vi "Create IMAQ Img from Channels.vi"(4 "Channel Name(s)":string[](array[string])) -> (0 "IMAQ Ch Images":T1[](array[typedef]), 1 "Channel Name(s) out":string[](array[string]))   [LabVIEW 2020]
uses:
  <vilib>/vision/Image Controls.llb/IMAQ Image.ctl
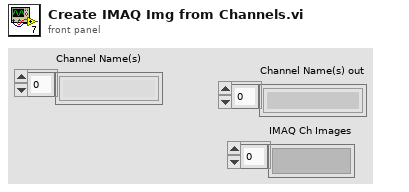
[diagram p1: front panel]
types:
  T1 = typedef "IMAQ Image.ctl" = refnum<image>
  T2 = typedef "Image Type" = u32
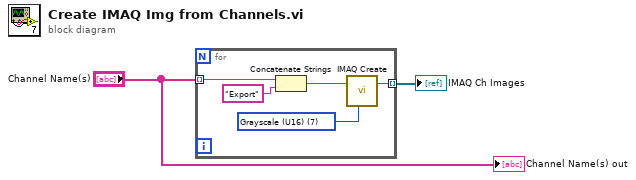
[diagram p0: block diagram]
diagram:
  n1 = for {
    tunnel: "Channel Name(s)" -> [w7] mode=indexing
    tunnel: [w3] -> w2 mode=indexing
    w5 = T2 7 items=["Grayscale (U8)", "Grayscale (I16)", "Grayscale (SGL)", "Complex (CSG)", "RGB (U32)", "HSL (U32)", "RGB (U64)", "Grayscale (U16)"] ("Image Type")
    n2 = Concatenate Strings(w7, "Export" ("string")) -> (w4:string)
    n3 = call "IMAQ Create"("Image Name"=w4, "Image Type"=w5) -> ("New Image"=w3:T1)  [unwired: 3 in, 1 out]
  }
  "IMAQ Ch Images" <- w2
  "Channel Name(s) out" <- "Channel Name(s)"
